vi "Set VISA.vi"(8 "error in (no error)":errorcluster, 10 "VISA":refnum<visa-resource-name>, 11 "Arduino Detector in":refnum<class "Arduino Detector.lvclass">) -> (0 "error out":errorcluster, 3 "Arduino Detector out":refnum<class "Arduino Detector.lvclass">)   [LabVIEW 2019, in "Arduino Detector.lvclass"]
uses:
  Arduino Detector.lvclass
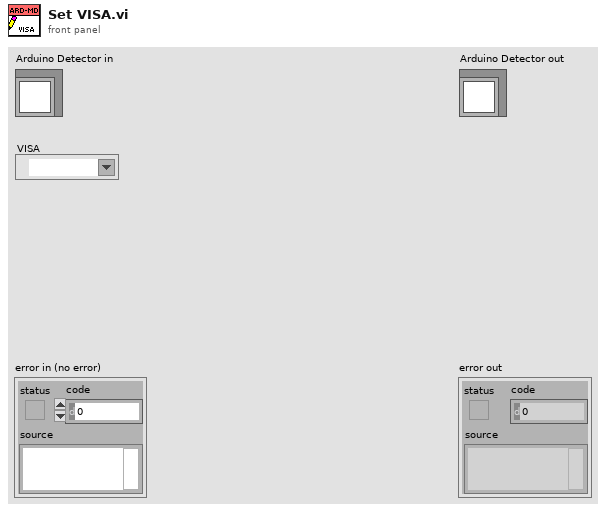
[diagram p1: front panel]
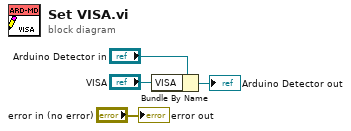
[diagram p0: block diagram]
diagram:
  n1 = Bundle By Name(cluster="Arduino Detector in", "VISA"="VISA") -> (→"Arduino Detector out":refnum<class "Arduino Detector.lvclass">)
  "error out" <- "error in (no error)"
